vi "XNET Reflective Memory Chan Page.vi"(8 "error in (no error)":errorcluster, 11 "Node Ptr":T3 format="%.0x") -> (0 "error out":errorcluster)   [LabVIEW 2010, in "XNET Reflective Memory Custom Device.lvlib"]
uses:
  XNET Reflective Memory Custom Device.lvlib
  <vilib>/NI Veristand/Custom Device API/Custom Device Item Ref.ctl
  ReadWrite.ctl
  BeforeAfter.ctl
  <vilib>/NI Veristand/Custom Device API/Custom Device Channel Type.ctl
  Global.vi
  <vilib>/NI Veristand/Custom Device API/Get Item Property (U16).vi
  <vilib>/NI VeriStand/Custom Device API/Set Item Property (U16).vi
  <vilib>/NI Veristand/Custom Device API/Custom Device API.lvlib
panel:
  in  "BeforeAfter?":T1 caption="Sync before or after model execution?"
  in  "ReadWrite?":T2 caption="Read or Write?"
  in  "Header":cluster{"Section Name":string}={"Section Name"="Custom Device Item Settings"}
  in  "Description":string
  in  "Name":string
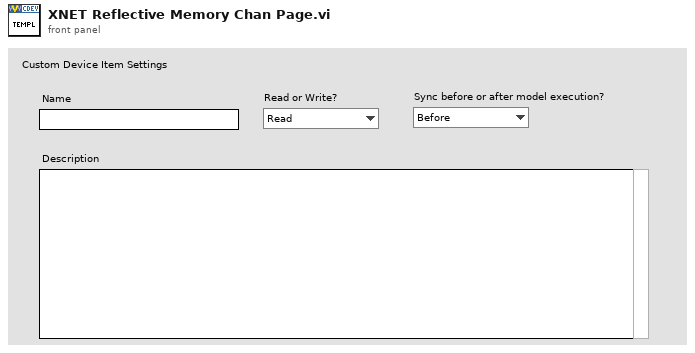
[diagram p1: front panel]
types:
  T1 = typedef "XNET Reflective Memory Custom Device.lvlib/BeforeAfter.ctl" = enum16{"Before", "After"}
  T2 = typedef "XNET Reflective Memory Custom Device.lvlib/ReadWrite.ctl" = enum16{"Read", "Write"}
  T3 = typedef "Custom Device API.lvlib/Custom Device Item Ref.ctl" = u64
  T4 = typedef "Custom Device API.lvlib/Custom Device Channel Type.ctl" = enum16{"Input", "Output"}
  T5 = typedef "Custom Device API.lvlib/Custom Device Channel.ctl" = cluster{"Type":T4, "Units":string, "Default Value":dbl, "Faultable":bool, "Scalable":bool}
  T6 = typedef "Custom Device API.lvlib/Custom Device Item Info.ctl" = cluster{"Name":string, "Is Channel":bool, "GUID":string}
  T7 = typedef "Custom Device API.lvlib/Custom Device Commands.ctl" = enum16{"Default", "Item renamed", "Shutdown", "Dynamic button pressed"}
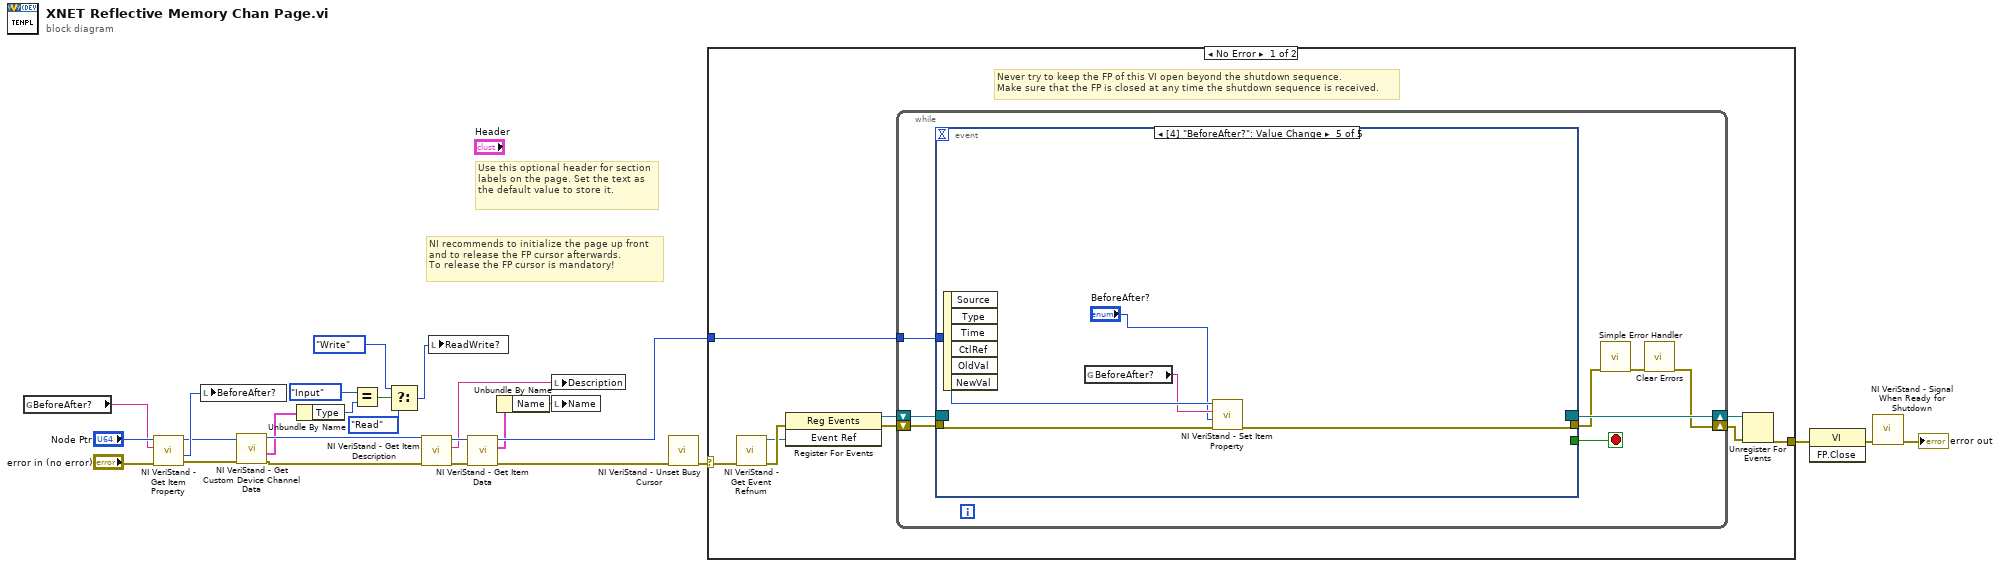
[diagram p0: block diagram]
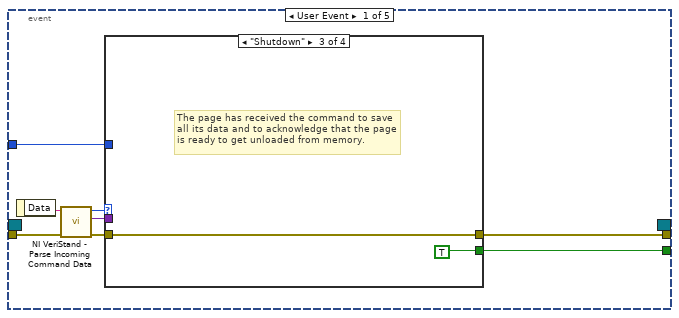
[diagram p2: hidden frame]
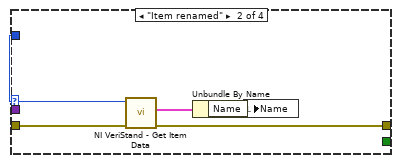
[diagram p4: hidden frame]
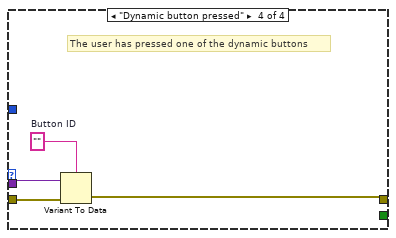
[diagram p5: hidden frame]
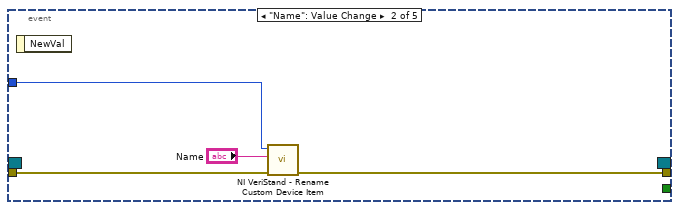
[diagram p6: hidden frame]
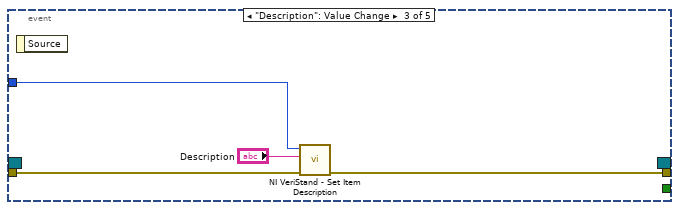
[diagram p7: hidden frame]
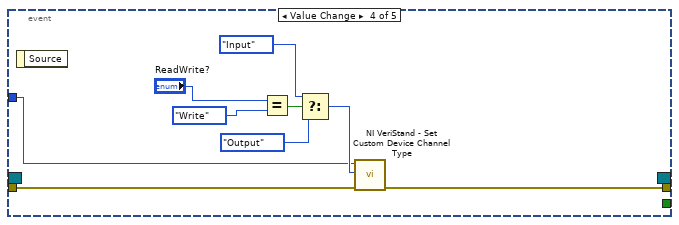
[diagram p8: hidden frame]
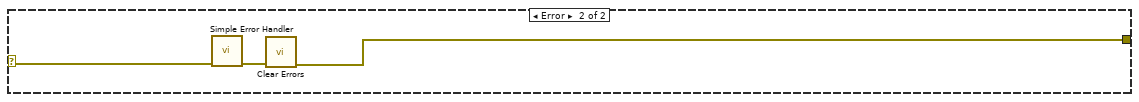
[diagram p9: hidden frame]
diagram:
  # "Use this optional header for section labels on the page. Set the text as the default value to store it."
  # "NI recommends to initialize the page up front\nand to release the FP cursor afterwards.\nTo release the FP cursor is mandatory!"
  n1 = global read "Global.vi" "BeforeAfter?"() -> (w13:string)
  n2 = call-poly <vilib>:"NI VeriStand - Get Item Property.vi"("error in (no error)"="error in (no error)", "Property Name"=w13, "Item Ref in"="Node Ptr") -> ("error out"=w1:errorcluster, "Value"=w12:u16, "Item Ref out"=w2:T3)  [unwired: 5 in, 1 out]
  n3 = local write "BeforeAfter?"(w12) -> ()
  n4 = call <vilib>:"NI VeriStand - Get Custom Device Channel Data.vi"("error in (no error)"=w1, "Channel Ref in"=w2) -> ("error out"=w11:errorcluster, "Channel"=w9:T5, "Channel Ref out"=w10:T3)  [unwired: 4 in, 3 out]
  n5 = Unbundle By Name(w9) -> ("Type"=w8:T4)
  n6 = Equal?(x=Custom_Device_Channel_Type."Input", y=w8) -> (x = y?=w6:bool)
  n7 = Select(t=ReadWrite."Write" ("ReadWrite?"), s=w6, f=ReadWrite."Read") -> (s? t:f=w4:T2)
  n8 = call <vilib>:"NI VeriStand - Get Item Description.vi"("error in (no error)"=w11, "Item Ref in"=w10) -> ("error out"=w18:errorcluster, "Description"=w19:string, "Item Ref out"=w20:T3)  [unwired: 7 out]
  n9 = local write "ReadWrite?"(w4) -> ()
  n10 = call <vilib>:"NI VeriStand - Get Item Data.vi"("error in (no error)"=w18, "Item Ref in"=w20) -> ("error out"=w23:errorcluster, "Item Info"=w17:T6, "Item Ref out"=w21:T3)  [unwired: 7 out]
  n11 = Unbundle By Name(w17) -> ("Name"=w16:string)
  n12 = local write "Description"(w19) -> ()
  n13 = local write "Name"(w16) -> ()
  n14 = call <vilib>:"NI VeriStand - Unset Busy Cursor.vi"("error in (no error)"=w23) -> ("error out"=w22:errorcluster)  [unwired: 10 out]
  n15 = case shown="No Error" w22 {
    selector: w22 -> [w27 w88]
    tunnel: [w32 w86] -> w26
    tunnel: w21 -> [w28 _]
    frame No Error {
      # "Never try to keep the FP of this VI open beyond the shutdown sequence.\nMake sure that the FP is closed at any time the shutdown sequence is received."
      n16 = call <vilib>:"NI VeriStand - Get Event Refnum.vi"("error in (no error)"=w27) -> ("error out"=w35:errorcluster, "Event Ref"=w31:refnum<user-event>)  [unwired: 9 out]
      n17 = register-events(error in=w35, w31) -> (reference out=w29:refnum<event-registration>, error out=w30:errorcluster)  [unwired: 1 in]
      n18 = while {
        tunnel: w28 -> [w39]
        shift-right: [w36] -> w33
        shift-left: w30 -> [w42]
        shift-right: [w43] -> w34
        shift-left: w29 -> [w41]
        stop <- w40 stop-if-true
        n19 = event shown="[4] \"BeforeAfter?\": Value Change" {
          selector: w41 -> [_ _ _ _ _]
          dyn-events: [_ _ _ _ _] -> w43
          timeout: _ -> [_ _ _ _ _]
          tunnel: w42 -> [w51 w67 w70 w80 w85]
          tunnel: [w47 _ _ _ _] -> w40
          tunnel: [w46 w66 w69 w72 w82] -> w38
          tunnel: w39 -> [w45 w65 w71 w73 w84]
          event User Event {
            n20 = event-data() -> ("Data"=w50:string)  [unwired: 1 out]
            n21 = call <vilib>:"NI VeriStand - Parse Incoming Command Data.vi"("error in (no error)"=w51, "Data"=w50) -> ("error out"=w49:errorcluster, "Data"=w44:variant, "Action"=w48:T7)  [unwired: 7 out]
            n22 = case shown="\"Shutdown\"" w48 {
              tunnel: w49 -> [w52 w57 w58 w63]
              tunnel: [_ _ TRUE _] -> w47
              tunnel: [w52 w54 w58 w60] -> w46
              tunnel: w45 -> [_ w56 _ _]
              tunnel: w44 -> [_ _ _ w62]
              frame "Default", Default {
              }
              frame "Item renamed" {
                n23 = call <vilib>:"NI VeriStand - Get Item Data.vi"("error in (no error)"=w57, "Item Ref in"=w56) -> ("error out"=w54:errorcluster, "Item Info"=w55:T6)  [unwired: 8 out]
                n24 = Unbundle By Name(w55) -> ("Name"=w53:string)
                n25 = local write "Name"(w53) -> ()
              }
              frame "Shutdown" {
                # "The page has received the command to save all its data and to acknowledge that the page is ready to get unloaded from memory."
              }
              frame "Dynamic button pressed" {
                w61 = ""  # Button ID
                # "The user has pressed one of the dynamic buttons"
                n26 = Variant To Data(error in=w63, Variant=w62, type=w61) -> (error out=w60:errorcluster)  [unwired: 1 out]
              }
            }
          }
          event "Name": Value Change {
            n27 = event-data() -> ()  [unwired: 2 out]
            n28 = call <vilib>:"NI VeriStand - Rename Custom Device Item.vi"("error in (no error)"=w67, "New Name"="Name", "Item Ref in"=w65) -> ("error out"=w66:errorcluster)  [unwired: 8 out]
          }
          event "Description": Value Change {
            n29 = event-data() -> ()  [unwired: 2 out]
            n30 = call <vilib>:"NI VeriStand - Set Item Description.vi"("error in (no error)"=w70, "Description"="Description", "Item Ref in"=w71) -> ("error out"=w69:errorcluster)  [unwired: 8 out]
          }
          event Value Change {
            n31 = event-data() -> ()  [unwired: 2 out]
            n32 = Equal?(x="ReadWrite?", y=ReadWrite."Write") -> (x = y?=w79:bool)
            n33 = Select(t=Custom_Device_Channel_Type."Input" ("Type"), s=w79, f=Custom_Device_Channel_Type."Output") -> (s? t:f=w74:T4)
            n34 = call <vilib>:"NI VeriStand - Set Custom Device Channel Type.vi"("error in (no error)"=w80, "Type"=w74, "Channel Ref in"=w73) -> ("error out"=w72:errorcluster)  [unwired: 7 in, 1 out]
          }
          event Value Change {
            n35 = event-data() -> ()  [unwired: 7 out]
            n36 = global read "Global.vi" "BeforeAfter?"() -> (w83:string)
            n37 = call-poly <vilib>:"NI VeriStand - Set Item Property.vi"("error in (no error)"=w85, "Value"="BeforeAfter?", "Property Name"=w83, "Item Ref in"=w84) -> ("error out"=w82:errorcluster)  [unwired: 5 in, 2 out]
          }
        }
        n38 = call <vilib>:"Simple Error Handler.vi"("error in (no error)"=w38) -> ("error out"=w37:errorcluster)  [unwired: 1 in, 7 out]
        n39 = call <vilib>:"Clear Errors.vi"("error in (no error)"=w37) -> ("error out"=w36:errorcluster)  [unwired: 6 out]
      }
      n40 = Unregister For Events(event registration refnum=w34, error in=w33) -> (error out=w32:errorcluster)
    }
    frame Error {
      n41 = call <vilib>:"Simple Error Handler.vi"("error in (no error)"=w88) -> ("error out"=w87:errorcluster)  [unwired: 1 in, 7 out]
      n42 = call <vilib>:"Clear Errors.vi"("error in (no error)"=w87) -> ("error out"=w86:errorcluster)  [unwired: 6 out]
    }
  }
  n43 = invoke class="VI" method="FP.Close"(error in=w26) -> (error out=w25:errorcluster)  [unwired: 2 in, 2 out]
  n44 = call <vilib>:"NI VeriStand - Signal When Ready for Shutdown.vi"("error in (no error)"=w25) -> ("error out"=→"error out":errorcluster)  [unwired: 10 out]
